vi "Read All Actual Values From Log File.vi"(8 "Error In":errorcluster, 10 "Log":path, 11 "Test Data":T1[](array[typedef])) -> (0 "Error Out":errorcluster, 1 "System Time":dbl[](array[numeric]), 2 "Actual Values":dbl[][](array[numeric]), 3 "Test Data dup":T1[](array[typedef]))   [LabVIEW 2011]
uses:
  Controls/Test Column Data.ctl
  Channel path to TDMS Group and Channel.vi
  Find Index of Timestamps.vi
  <vilib>/Utility/error.llb/Error Cluster From Error Code.vi
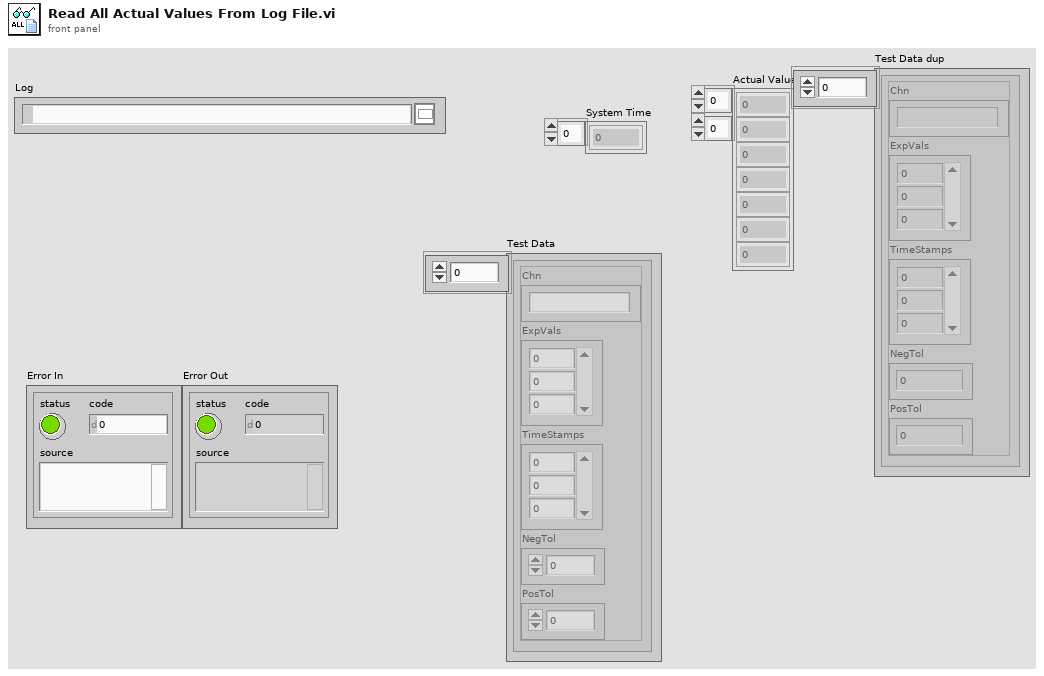
[diagram p1: front panel]
types:
  T1 = typedef "Test Column Data.ctl" = cluster{"Chn":string, "ExpVals":dbl[], "TimeStamps":i64[], "NegTol":dbl, "PosTol":dbl}
  T2 = enum16{"open", "open or create", "create or replace", "create", "open (read-only)"}
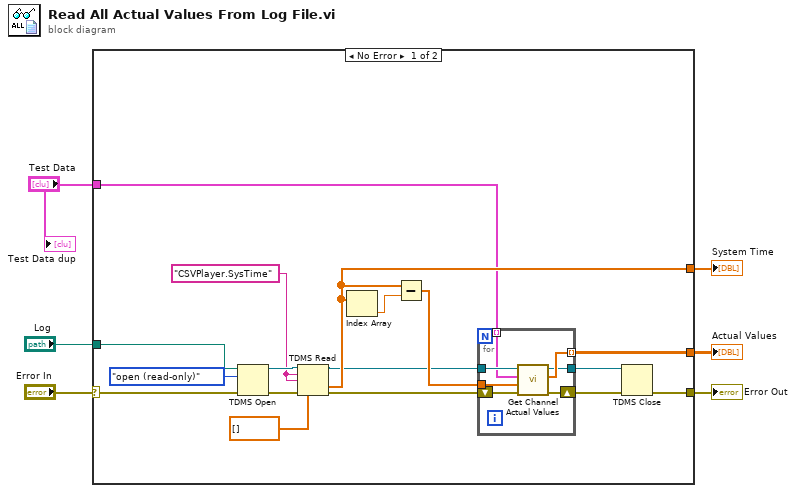
[diagram p0: block diagram]
diagram:
  n1 = case shown="No Error" "Error In" {
    selector: "Error In" -> [w13 w31]
    tunnel: "Log" -> [w23 _]
    tunnel: "Test Data" -> [w8 _]
    tunnel: [w14 w31] -> w5
    tunnel: [w12 _] -> w3
    tunnel: [w11 _] -> w2
    frame No Error {
      w20 = "CSVPlayer.SysTime" ("group name in")
      n2 = TDMS Open(8:w13, 10:T2."open (read-only)" ("operation (0:open)"), 11:w23) -> (0:w22:errorcluster, 3:w21:refnum<k34>)  [unwired: 3 in]
      n3 = TDMS Read(0:w21, 5:w20, 7:w20, 11:w22, 12:dbl[] []) -> (4:w10:refnum<k34>, 10:w11:dbl[], 15:w17:errorcluster)  [unwired: 3 in, 3 out]
      n4 = Index Array(array=w11) -> (element=w19:dbl)  [unwired: 1 in]
      n5 = Subtract(x=w11, y=w19) -> (x-y=w18:dbl[])
      n6 = for {
        tunnel: w18 -> [w30]
        tunnel: [w27] -> w12 mode=indexing
        shift-right: [w28] -> w15
        shift-left: w17 -> [w29]
        tunnel: w10 -> [w26]
        tunnel: [w25] -> w9
        tunnel: w8 -> [w24] mode=indexing
        n7 = call "Get Channel Actual Values.vi"("error in (no error)"=w29, "System Time"=w30, "Column Data"=w24, "TDMS in"=w26) -> ("error out"=w28:errorcluster, "Actual Values"=w27:dbl[], "TDMS Out"=w25:refnum<k34>)  [unwired: 5 in]
      }
      n8 = TDMS Close(8:w15, 11:w9) -> (0:w14:errorcluster)  [unwired: 1 out]
    }
    frame Error {
    }
  }
  "Error Out" <- w5
  "Actual Values" <- w3
  "System Time" <- w2
  "Test Data dup" <- "Test Data"
